vi "Read Parameter from Word.vi"(8 "error in":errorcluster, 9 "parameter definition":T1={"start index"=10, "size"=19, "encoding"=enum."BNR", "signed"=FALSE, "scale multiplier"=1.0, "scale offset"=0.0}, 11 "ARINC 429 in":refnum<class "ARINC 429.lvclass">) -> (0 "error out":errorcluster, 2 "parameter value":dbl, 3 "ARINC 429 out":refnum<class "ARINC 429.lvclass">)   [LabVIEW 2020, in "ARINC 429.lvclass"]
uses:
  ARINC 429.lvclass
  Parameter Definition.ctl
  <vilib>/addons/VeriStand Custom Device Scripting APIs/Ballard ARINC 429/Encoding and Decoding/Encoding.ctl
  <vilib>/addons/VeriStand Custom Device Scripting APIs/Ballard ARINC 429/Encoding and Decoding/Encoding and Decoding.lvlib
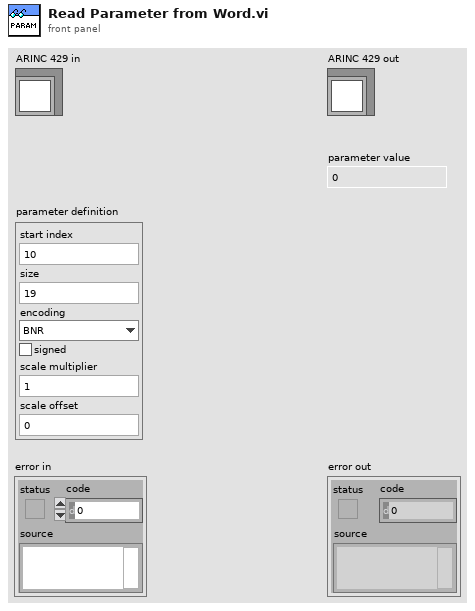
[diagram p1: front panel]
types:
  T1 = typedef "ARINC 429.lvclass/Parameter Definition.ctl" = cluster{"start index":i32, "size":i32, "encoding":T2, "signed":bool, "scale multiplier":dbl, "scale offset":dbl}
  T2 = typedef "Encoding and Decoding.lvlib/Encoding.ctl" = enum16{"BNR", "BCD", "Discrete"}
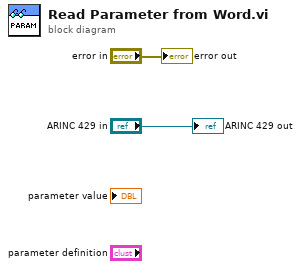
[diagram p0: block diagram]
diagram:
  "error out" <- "error in"
  "ARINC 429 out" <- "ARINC 429 in"
